vi "Destroy.vi"(0 "reference":refnum<class "StateNode.lvclass">, 5 "error in (no error)":errorcluster) -> (14 "reference out":refnum<class "StateNode.lvclass">, 19 "error out":errorcluster)   [LabVIEW 2016, in "StateNode.lvclass"]
doc: "Destroys a StateNode object created with a StateNode constructor VI.\n\n[GOOP 2.1]"
uses:
  <resource>/Framework/Providers/Open_GDS/UML/StateNode_class/StateNode.lvclass
  <resource>/Framework/Providers/Open_GDS/UML/RectangularNode_class/RectangularNode.lvclass
  <resource>/Framework/Providers/Open_GDS/UML/MultiLineString_class/MultiLineString.lvclass
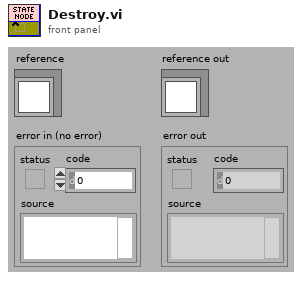
[diagram p1: front panel]
types:
  T1 = typedef "StateNode.lvclass/ObjectAttributes.ctl" = cluster{"state":refnum<class "MultiLineString.lvclass">, "action":refnum<class "MultiLineString.lvclass">, "DEFAULT_WIDTH":i32, "DEFAULT_HEIGHT":i32}
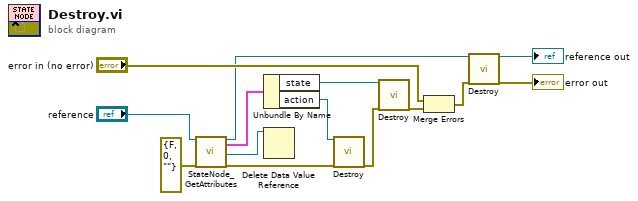
[diagram p0: block diagram]
diagram:
  n1 = call <resource>:"StateNode_GetAttributes.vi"("reference in"="reference", "error in (no error)"=errorcluster {"status"=FALSE, "code"=0, "source"=""}) -> ("reference out"=w5:refnum<class "StateNode.lvclass">, "Data"=w3:T1, "DataRef"=w2:refnum<data-value>, "error out"=w7:errorcluster)  [unwired: 1 in, 13 out]
  n2 = Unbundle By Name(w3) -> ("state"=w10:refnum<class "MultiLineString.lvclass">, "action"=w6:refnum<class "MultiLineString.lvclass">)
  n3 = Delete Data Value Reference(data value reference=w2) -> ()  [unwired: 1 in, 2 out]
  n4 = call-dynamic "Destroy.vi"("reference"=w6, "error in (no error)"=w7) -> ("error out"=w8:errorcluster)  [unwired: 16 in, 1 out]
  n5 = call-dynamic "Destroy.vi"("reference"=w10, "error in (no error)"=w8) -> ("error out"=w9:errorcluster)  [unwired: 16 in, 1 out]
  n6 = Merge Errors("error in (no error)", w9) -> (w4:errorcluster)
  n7 = call-parent "Destroy.vi"("reference"=w5, "error in (no error)"=w4) -> ("reference out"=→"reference out":refnum<class "StateNode.lvclass">, "error out"=→"error out":errorcluster)  [unwired: 16 in]
